vi "GFGbooleanGet.vi"(7 "GFG Refnum (use when calling from external project)":refnum<vi>, 11 "Variable Name in":string) -> (2 "Found/Replaced":bool, 3 "Boolean Value OUT":bool)   [LabVIEW 2017, in "GFG library.lvlib"]
doc: "SciScan 1.2 160622"
uses:
  GFG library.lvlib
panel:
  in  "error in (no error)":errorcluster
  out "error out":errorcluster
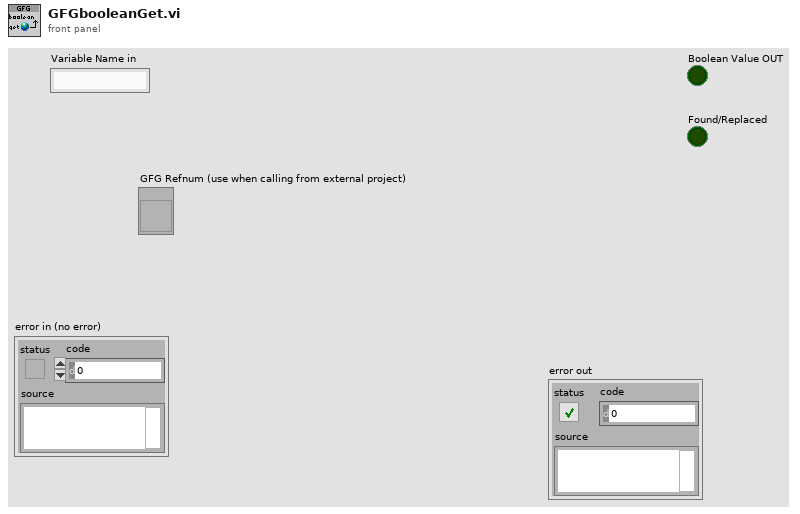
[diagram p1: front panel]
types:
  T1 = typedef "VariantType.lvlib/Type.ctl" = enum8{"Invalid Type", "Void", "I8", "I16", "I32", "I64", "U8", "U16", "U32", "U64", "Single Float", "Double Float", "Extended Float", "Single Complex", "Double Complex", "Extended Complex", "Enum U8", "Enum U16", "Enum U32", "Enum U64", "Single Float With Unit", "Double Float With Unit", "Extended Float With Unit", "Single Complex with Unit", "Double Complex with Unit", "Extended Complex with Unit", "Boolean", "String", "Path", "Picture", "Tag", "Array", "Cluster", "Variant", "LV Variant", "Waveform", "Timestamp", "Digital Waveform", "Digital Data", "ExpressData", "Refnum", "External Data", "VI", "Poly VI", "LabVIEW Class Instance", "Fixed Point"}
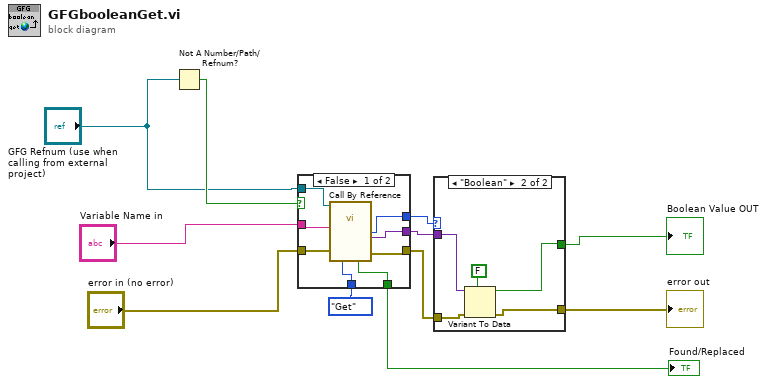
[diagram p0: block diagram]
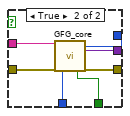
[diagram p2: hidden frame]
diagram:
  n1 = Not A Number/Path/Refnum?(number/path/refnum="GFG Refnum (use when calling from external project)") -> (NaN/Path/Refnum?=w8:bool)
  n2 = case shown="False" w8 {
    tunnel: enum16{"Init", "Set", "Get"}."Get" ("Action") -> [w14 w26]
    tunnel: "Variable Name in" -> [w15 w25]
    tunnel: "error in (no error)" -> [w19 w24]
    tunnel: [w18 w23] -> w4
    tunnel: [w16 w22] -> w5
    tunnel: [w17 w21] -> w6
    tunnel: "GFG Refnum (use when calling from external project)" -> [w13 _]
    tunnel: [w12 w20] -> w1
    frame False {
      n3 = call-by-ref "?"(reference=w13, "Variable Name in"=w15, "error in (no error)"=w19, "Action"=w14) -> ("Found/Replaced"=w12:bool, "Data Type Out"=w16:T1, "Variant Out"=w17:variant, "error out"=w18:errorcluster)  [unwired: 11 in, 5 out]
    }
    frame True {
      n4 = call "GFG_core.vi"("Variable Name in"=w25, "error in (no error)"=w24, "Action"=w26) -> ("Found/Replaced"=w20:bool, "Data Type Out"=w22:T1, "Variant Out"=w21:variant, "error out"=w23:errorcluster)  [unwired: 10 in, 3 out]
    }
  }
  "Found/Replaced" <- w1
  n5 = case shown="\"Boolean\"" w5 {
    tunnel: w6 -> [_ w32]
    tunnel: [_ w30] -> w11
    tunnel: w4 -> [w27 w29]
    tunnel: [w27 w28] -> w10
    frame Default {
    }
    frame "Boolean" {
      n6 = Variant To Data(error in=w29, type=FALSE, Variant=w32) -> (data=w30:bool, error out=w28:errorcluster)
    }
  }
  "Boolean Value OUT" <- w11
  "error out" <- w10
